vi "Gnuplot_offset_ytics.vi"(1 "Separation":dbl=1.2, 2 "Mode":T1, 3 "precision":string, 4 "Legend":string[](array[string]), 5 "Max Plot Value":dbl, 6 "Profile offset":dbl) -> (0 "concatenated string":string)   [LabVIEW 2011]
uses:
  Gnuplot_Label.ctl
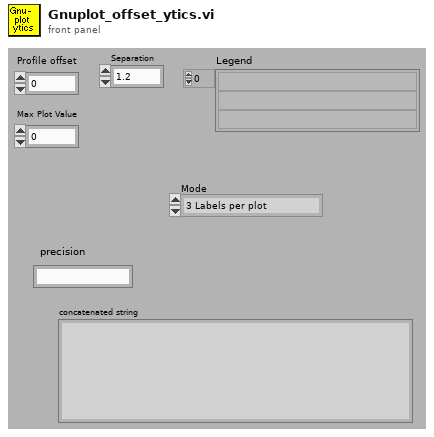
[diagram p1: front panel]
types:
  T1 = typedef "Gnuplot_Label.ctl" = enum16{"3 Labels per plot", "Only Center label", "Only Bottom Label"}
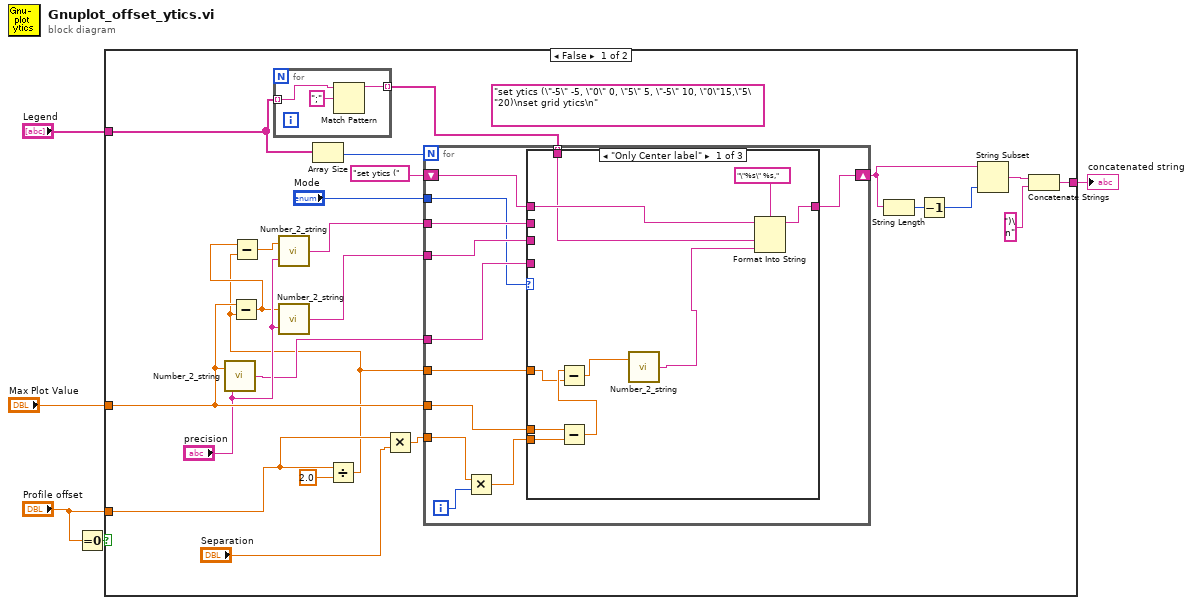
[diagram p0: block diagram]
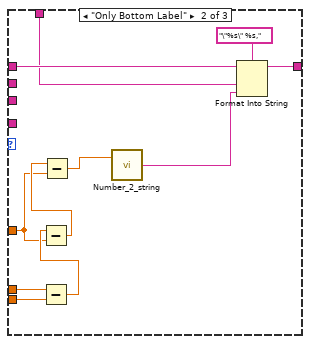
[diagram p2: hidden frame]
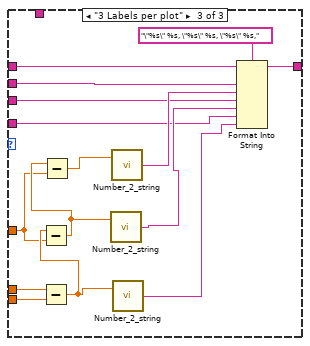
[diagram p3: hidden frame]
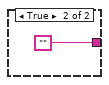
[diagram p4: hidden frame]
diagram:
  n1 = Equal To 0?(x="Profile offset") -> (x = 0?=w2:bool)
  n2 = case shown="False" w2 {
    tunnel: "Legend" -> [w7 _]
    tunnel: "Max Plot Value" -> [w27 _]
    tunnel: "Profile offset" -> [w14 _]
    tunnel: [w15 ""] -> w3
    frame False {
      (unwired) "set ytics (\"-5\" -5, \"0\" 0, \"5\" 5, \"-5\" 10, \"0\"15,\"5\"20)\nset grid ytics\n"
      n3 = call "Number_2_string.vi"("precision"="precision", "number"=w27) -> ("String"=w22:string)
      n4 = for {
        tunnel: w7 -> [w30] mode=indexing
        tunnel: [w29] -> w8 mode=indexing
        n5 = Match Pattern(string=w30, regular expression=";") -> (before substring=w29:string)  [unwired: 4 out]
      }
      n6 = Array Size(array=w7) -> (size(s)=w6:i32)
      n7 = Divide(x=w14, y=2.0) -> (x/y=w11:dbl)
      n8 = Subtract(x=w27, y=w11) -> (x-y=w12:dbl)
      n9 = Subtract(x=w12, y=w11) -> (x-y=w26:dbl)
      n10 = call "Number_2_string.vi"("precision"="precision", "number"=w26) -> ("String"=w24:string)
      n11 = call "Number_2_string.vi"("precision"="precision", "number"=w12) -> ("String"=w23:string)
      n12 = Multiply(x=w14, y="Separation") -> (x*y=w13:dbl)
      n13 = for {
        N: w6 -> [_]
        tunnel: w27 -> [w40]
        tunnel: w13 -> [w42]
        tunnel: w11 -> [w34]
        tunnel: w24 -> [w39]
        tunnel: w23 -> [w36]
        tunnel: w22 -> [w35]
        shift-right: [w37] -> w18
        shift-left: "set ytics (" ("format string") -> [w38]
        tunnel: "Mode" -> [w33]
        tunnel: w8 -> [w32] mode=indexing
        i -> [w43]
        n14 = Multiply(x=w42, y=w43) -> (x*y=w41:dbl)
        n15 = case shown="\"Only Center label\"" w33 {
          tunnel: w41 -> [w53 w64 w79]
          tunnel: w40 -> [w52 w63 w78]
          tunnel: w39 -> [_ _ w76]
          tunnel: w38 -> [w50 w60 w73]
          tunnel: [w49 w59 w72] -> w37
          tunnel: w36 -> [_ _ w71]
          tunnel: w35 -> [_ _ w69]
          tunnel: w34 -> [w45 w56 w65]
          tunnel: w32 -> [w44 w54 _]
          frame "Only Center label" {
            n16 = Subtract(x=w52, y=w53) -> (x-y=w47:dbl)
            n17 = Subtract(x=w47, y=w45) -> (x-y=w46:dbl)
            n18 = call "Number_2_string.vi"("number"=w46) -> ("String"=w48:string)  [unwired: 1 in]
            n19 = Format Into String(format string="\"%s\" %s,", initial string=w50, w44, w48) -> (resulting string=w49:string)  [unwired: 1 in, 1 out]
          }
          frame "Only Bottom Label" {
            n20 = Subtract(x=w63, y=w64) -> (x-y=w58:dbl)
            n21 = Subtract(x=w58, y=w56) -> (x-y=w57:dbl)
            n22 = Subtract(x=w57, y=w56) -> (x-y=w62:dbl)
            n23 = call "Number_2_string.vi"("number"=w62) -> ("String"=w55:string)  [unwired: 1 in]
            n24 = Format Into String(format string="\"%s\" %s,", initial string=w60, w54, w55) -> (resulting string=w59:string)  [unwired: 1 in, 1 out]
          }
          frame "3 Labels per plot" {
            n25 = Subtract(x=w78, y=w79) -> (x-y=w67:dbl)
            n26 = Subtract(x=w67, y=w65) -> (x-y=w66:dbl)
            n27 = Subtract(x=w66, y=w65) -> (x-y=w77:dbl)
            n28 = call "Number_2_string.vi"("number"=w66) -> ("String"=w70:string)  [unwired: 1 in]
            n29 = call "Number_2_string.vi"("number"=w77) -> ("String"=w75:string)  [unwired: 1 in]
            n30 = call "Number_2_string.vi"("number"=w67) -> ("String"=w68:string)  [unwired: 1 in]
            n31 = Format Into String(format string="\"%s\" %s, \"%s\" %s, \"%s\" %s,", initial string=w73, w76, w75, w71, w70, w69, w68) -> (resulting string=w72:string)  [unwired: 1 in, 1 out]
          }
        }
      }
      n32 = String Length(string=w18) -> (length=w20:i32)
      n33 = Decrement(x=w20) -> (x-1=w19:i32)
      n34 = String Subset(string=w18, length (rest)=w19) -> (substring=w17:string)  [unwired: 1 out]
      n35 = Concatenate Strings(w17, ")\n" ("string")) -> (w15:string)
    }
    frame True {
    }
  }
  "concatenated string" <- w3
